vi "Send Set Response to Error.vi"(7 "Message Priority (Normal)":T2=enum."Normal", 8 "error in (no error)":errorcluster, 10 "response":T1, 11 "Message Enqueuer":refnum<class "Message Enqueuer.lvclass">) -> (0 "error out":errorcluster, 3 "Message Enqueuer out":refnum<class "Message Enqueuer.lvclass">)   [LabVIEW 2021, in "Error Handler.lvlib" / "Set Response to Error Msg.lvclass"]
doc: "This VI sends the message to an actor."
uses:
  Set Response to Error Msg.lvclass
  <vilib>/ActorFramework/Message Enqueuer/Message Enqueuer.lvclass
  <vilib>/ActorFramework/Message Enqueuer/Message Priority.ctl
  public types/response.ctl
  C:/Program Files (x86)/National Instruments/LabVIEW 2021/vi.lib/ActorFramework/Message/Message.lvclass
  Set Response to Error Msg.lvclass/Set Response to Error Msg.ctl
  <vilib>/ActorFramework/Message Enqueuer/Message Enqueuer.lvclass/Message Enqueuer.ctl
  <vilib>/ActorFramework/Message Priority Queue/Priority Enqueue.vi
  C:/Repositories/LabVIEW/Actor/Actor-Dice-Game/src/Actors/Error Handler/Error Handler Messages/Set Response to Error Msg/Set Response to Error Msg.lvclass
  Error Handler.lvlib
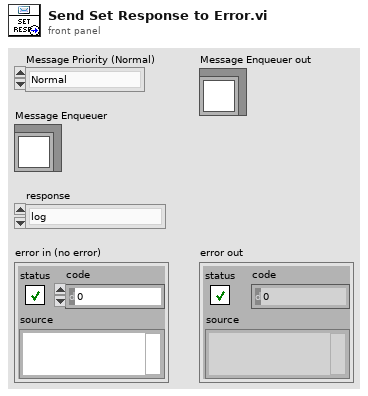
[diagram p1: front panel]
types:
  T1 = typedef "Error Handler.lvlib/response.ctl" = enum16{"log", "log & popup", "log & exit", "log & popup & exit", "popup", "popup & exit", "exit", "ignore"}
  T2 = typedef "Actor Framework.lvlib/Message Enqueuer.lvclass/Message Priority.ctl" = enum16{"Low", "Normal", "High"}
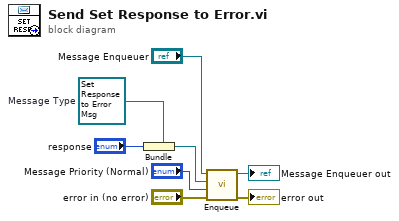
[diagram p0: block diagram]
diagram:
  w5 = refnum<class "Set Response to Error Msg.lvclass"> refnum  # Message Type
  n1 = Bundle(cluster=w5, "response") -> (w4:refnum<class "Set Response to Error Msg.lvclass">)
  n2 = call <vilib>:"Enqueue.vi"("error in (no error)"="error in (no error)", "Message Priority (Normal)"="Message Priority (Normal)", "Message"=w4, "Message Enqueuer in"="Message Enqueuer") -> ("error out"=→"error out":errorcluster, "Message Enqueuer in"=→"Message Enqueuer out":refnum<class "Message Enqueuer.lvclass">)  [unwired: 6 in]
